vi "sequence on all execution systems.vi"() -> ()   [LabVIEW 2015]
uses:
  result/result.lvclass
  dispatcher/pool sizes.ctl
  result/result.lvclass/result.ctl
  result/get data.vi
  result/get error.vi
  result/get owning task.vi
  result/get subresults.vi
  task/task.lvclass
  dispatcher/thread pool.lvclass
  standard reporters/event reporter/event reporter.lvclass
  standard tasks/sequence task/sequence task.lvclass
  standard action/wait action/wait action.lvclass
panel:
  out "logical AND":bool
  out "times":u32[](array[numeric])
  out "error":errorcluster
  out "data":variant
  out "accessors:subresults":refnum<class "result.lvclass">[][](array[class])
  out "Array 2":errorcluster[](array[cluster])
  out "Array":variant[](array[variant])
  out "Time":u32
  out "result":refnum<class "result.lvclass">
  out "error out":errorcluster
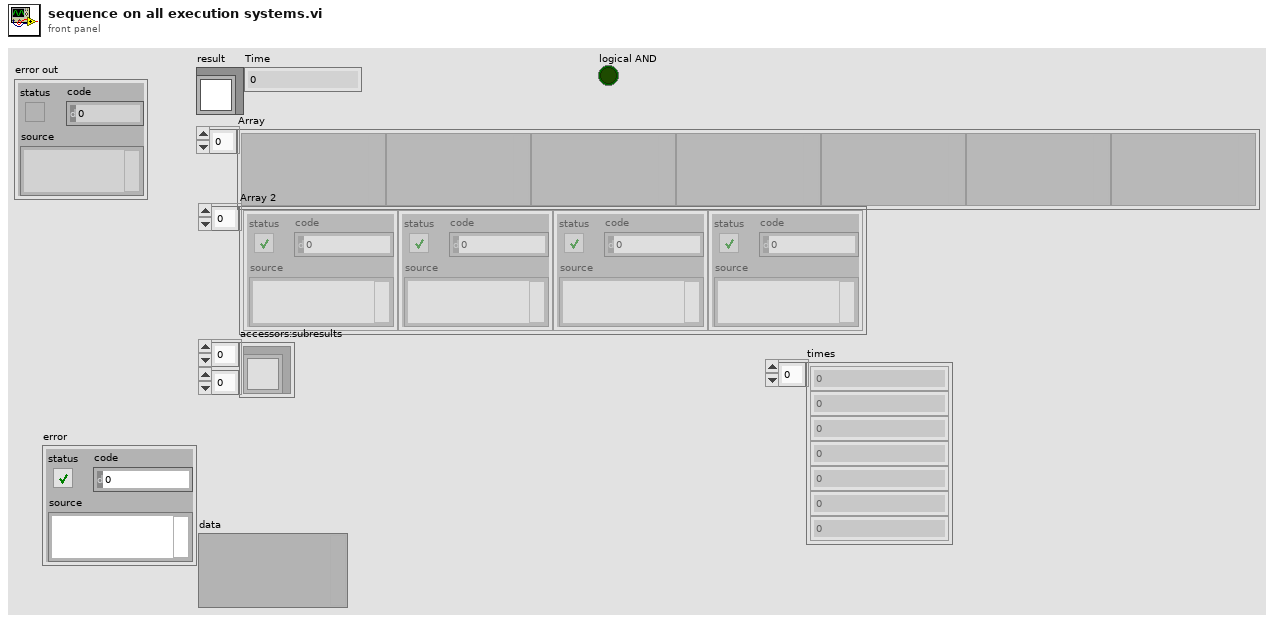
[diagram p1: front panel]
types:
  T1 = typedef "thread pool.lvclass/pool sizes.ctl" = cluster{"UI thread":u8, "standard":u8, "instrument I/O":u8, "data acquisition":u8, "other 1":u8, "other 2":u8}
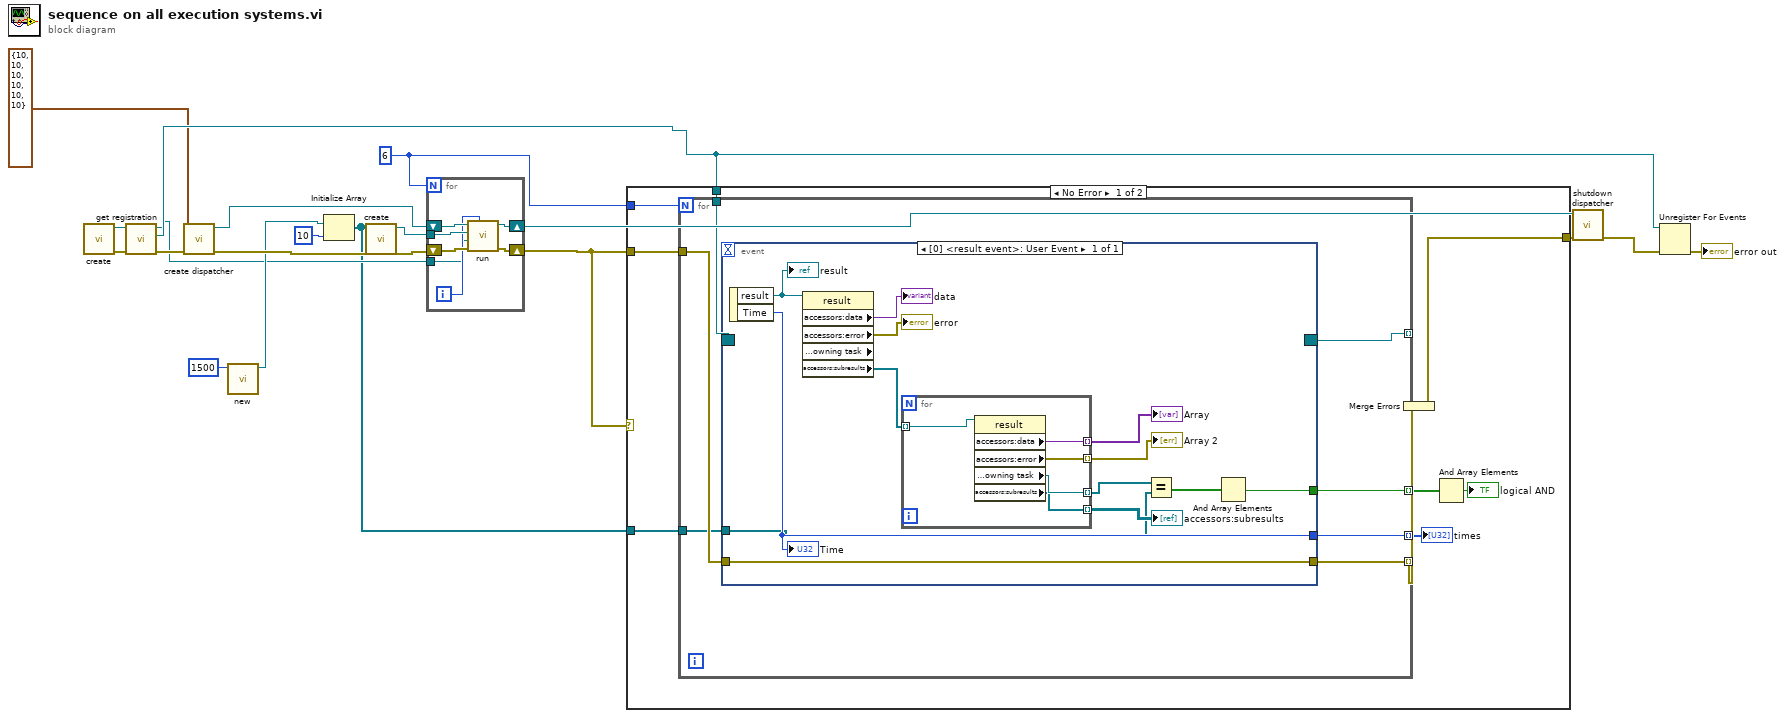
[diagram p0: block diagram]
diagram:
  w7 = 6
  n1 = call "create.vi"() -> ("error out"=w16:errorcluster, "event reporter out"=w17:refnum<class "event reporter.lvclass">)  [unwired: 10 in]
  n2 = call "get registration.vi"("error in"=w16, "event reporter in"=w17) -> ("error out"=w15:errorcluster, "result registration"=w8:refnum<event-registration>, "event reporter out"=w2:refnum<class "event reporter.lvclass">)  [unwired: 7 in]
  n3 = call "create dispatcher.vi"("error in"=w15, "pool sizes (standard=10)"=T1 {"UI thread"=10, "standard"=10, "instrument I/O"=10, "data acquisition"=10, "other 1"=10, "other 2"=10} ("initial pool sizes")) -> ("error out"=w18:errorcluster, "dispatcher"=w19:refnum<class "thread pool.lvclass">)  [unwired: 8 in]
  n4 = call "new.vi"("timer"=1500) -> ("wait action out"=w3:refnum<class "wait action.lvclass">)  [unwired: 10 in]
  n5 = Initialize Array(w3, 10 ("dimension size")) -> (w1:refnum<class "wait action.lvclass">[])
  n6 = call "create.vi"("tasks"=w1) -> ("sequence task out"=w10:refnum<class "sequence task.lvclass">)  [unwired: 10 in]
  n7 = for {
    N: w7 -> [_]
    tunnel: w10 -> [w23]
    shift-right: [w25] -> w14
    shift-left: w19 -> [w26]
    shift-right: [w24] -> w6
    shift-left: w18 -> [w22]
    tunnel: w2 -> [w20]
    i -> [w21]
    n8 = call "run.vi"("execution system"=w21, "error in"=w22, "results reporter"=w20, "task"=w23, "thread pool in"=w26) -> ("error out"=w24:errorcluster, "thread pool out"=w25:refnum<class "thread pool.lvclass">)  [unwired: 5 in]
  }
  n9 = case shown="No Error" w6 {
    tunnel: w6 -> [w35 w61]
    tunnel: [w33 w61] -> w9
    tunnel: w8 -> [w32 _]
    tunnel: w7 -> [w31 _]
    tunnel: w1 -> [w29 _]
    frame No Error {
      n10 = for {
        N: w31 -> [_]
        tunnel: w32 -> [w42]
        tunnel: [w41] -> _ mode=indexing
        tunnel: [w40] -> w34 mode=indexing
        tunnel: w35 -> [w39]
        tunnel: [w38] -> w30 mode=indexing
        tunnel: w29 -> [w37]
        tunnel: [w36] -> w28 mode=indexing
        n11 = event shown="[0] <result event>: User Event" {
          selector: w42 -> [_]
          dyn-events: [_] -> w41
          timeout: _ -> [_]
          tunnel: [w55] -> w40
          tunnel: w39 -> [w55]
          tunnel: [w47] -> w38
          tunnel: w37 -> [w45]
          tunnel: [w44] -> w36
          event User Event {
            n12 = event-data() -> ("result"=w54:refnum<class "result.lvclass">, "Time"=w47:u32)  [unwired: 1 in]
            "result" <- w54
            "Time" <- w47
            n13 = property class="result" props=["accessors:data", "accessors:error", "accessors:owning task", "accessors:subresults"](reference=w54) -> ("accessors:data"=→"data":variant, "accessors:error"=→"error":errorcluster, "accessors:subresults"=w53:refnum<class "result.lvclass">[])  [unwired: 1 in, 3 out]
            n14 = for {
              tunnel: w53 -> [w60] mode=indexing
              tunnel: [w59] -> w52 mode=indexing
              tunnel: [w58] -> w51 mode=indexing
              tunnel: [w57] -> w46 mode=indexing
              tunnel: [w56] -> w50 mode=indexing
              n15 = property class="result"(reference=w60) -> ("accessors:data"=w59:variant, "accessors:error"=w58:errorcluster, "accessors:owning task"=w57:refnum<class "task.lvclass">, "accessors:subresults"=w56:refnum<class "result.lvclass">[])  [unwired: 1 in, 2 out]
            }
            "Array" <- w52
            "Array 2" <- w51
            "accessors:subresults" <- w50
            n16 = Equal?(x=w46, y=w45) -> (x = y?=w43:bool[])
            n17 = And Array Elements(Boolean array=w43) -> (logical AND=w44:bool)
          }
        }
      }
      "times" <- w30
      n18 = Merge Errors(w34) -> (w33:errorcluster)
      n19 = And Array Elements(Boolean array=w28) -> (logical AND=→"logical AND":bool)
    }
    frame Error {
    }
  }
  n20 = call "shutdown dispatcher.vi"("error in"=w9, "thread pool"=w14) -> ("error out"=w13:errorcluster)  [unwired: 9 in]
  n21 = Unregister For Events(event registration refnum=w8, error in=w13) -> (error out=→"error out":errorcluster)
